vi "SignalAttrbGet_Reorder.vi"(0 "MessageFrame":refnum<k21>="ESP_1\nLRA110") -> (12 "SignalArryOderByStartBit":refnum<k21>[](array[refnum]), 14 "SignalsNameArry":string[](array[string]), 15 "ScaleFac":dbl[](array[numeric]), 16 "StartBitArry":u32[](array[numeric]), 17 "Length":u32[](array[numeric]), 18 "DataType":u32[](array[numeric]), 19 "DefaultValue":dbl[](array[numeric]))   [LabVIEW 2020]
uses:
  <resource>/objmgr/xnet.rc
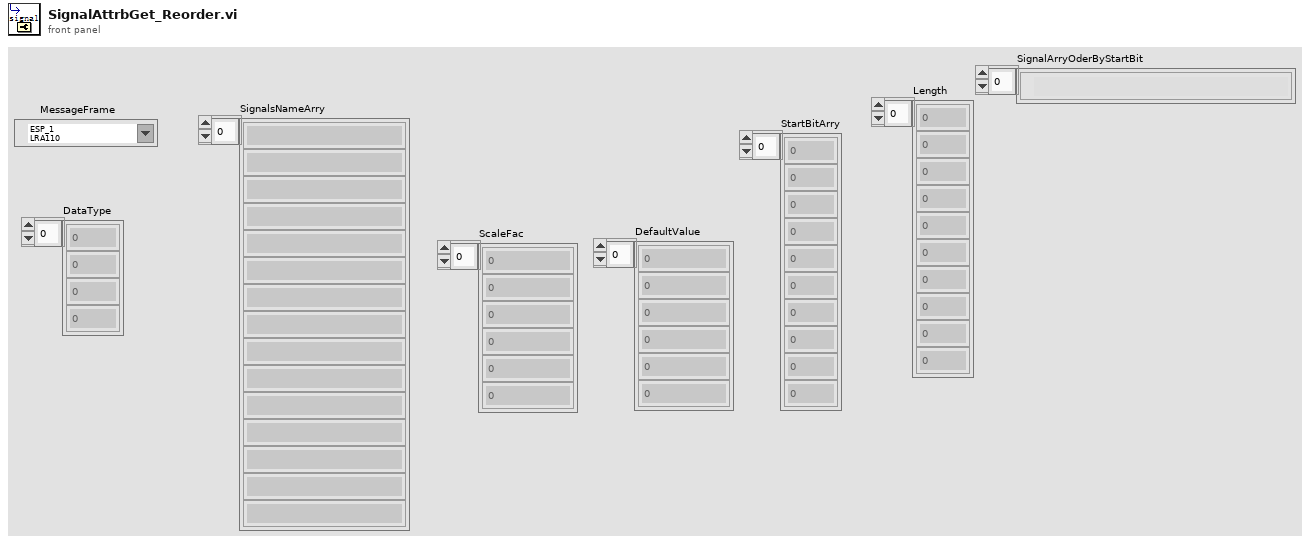
[diagram p1: front panel]
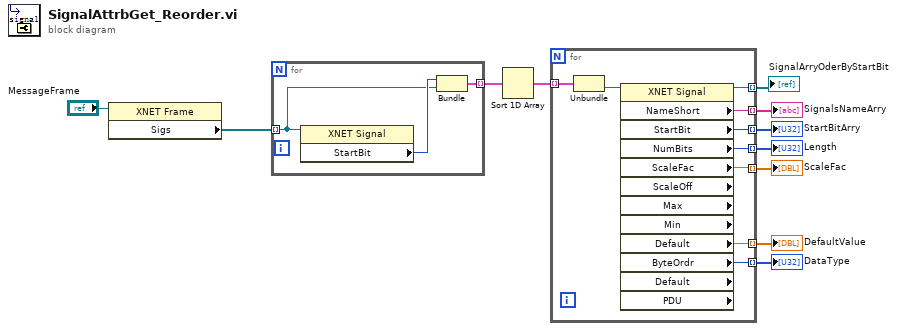
[diagram p0: block diagram]
diagram:
  n1 = property class="XNET Frame"(reference="MessageFrame") -> ("Sigs"=w2:refnum<k21>[])  [unwired: 1 in, 2 out]
  n2 = for {
    tunnel: w2 -> [w13] mode=indexing
    tunnel: [w12] -> w10 mode=indexing
    n3 = property class="XNET Signal"(reference=w13) -> ("StartBit"=w14:u32)  [unwired: 1 in, 2 out]
    n4 = Bundle("StartBit"=w14, w13) -> (w12:cluster{"StartBit":u32, refnum<k21>})  [unwired: 1 in]
  }
  n5 = Sort 1D Array(array=w10) -> (sorted array=w9:cluster{"StartBit":u32, refnum<k21>}[])
  n6 = for {
    tunnel: [w23] -> w8 mode=indexing
    tunnel: [w22] -> w5 mode=indexing
    tunnel: [w21] -> w4 mode=indexing
    tunnel: [w18] -> w7 mode=indexing
    tunnel: [w20] -> w3 mode=indexing
    tunnel: [w19] -> w6 mode=indexing
    tunnel: w9 -> [w17] mode=indexing
    tunnel: [w15] -> w1 mode=indexing
    n7 = Unbundle(w17) -> (w16:refnum<k21>)  [unwired: 1 out]
    n8 = property class="XNET Signal" props=["NameShort", "StartBit", "NumBits", "ScaleFac", "ScaleOff", "Max", "Min", "Default", "ByteOrdr", "Default", "PDU"](reference=w16) -> (reference out=w15:refnum<k21>, "NameShort"=w23:string, "StartBit"=w18:u32, "NumBits"=w19:u32, "ScaleFac"=w22:dbl, "Default"=w21:dbl, "ByteOrdr"=w20:u32)  [unwired: 1 in, 6 out]
  }
  "SignalsNameArry" <- w8
  "ScaleFac" <- w5
  "DefaultValue" <- w4
  "StartBitArry" <- w7
  "DataType" <- w3
  "Length" <- w6
  "SignalArryOderByStartBit" <- w1
